vi "TriggerAndAveraging.vi"(7 "Channel":i32, 8 "error in (no error)":errorcluster, 11 "C4209 PNA":refnum<class "C4209 PNA.lvclass">) -> (0 "error out":errorcluster, 3 "C4209 PNA out":refnum<class "C4209 PNA.lvclass">)   [LabVIEW 2017, in "C4209 PNA.lvclass"]
uses:
  C4209 PNA.lvclass
  C4209 PNA.lvclass/C4209 PNA.ctl
  <instrlib>/CMT S2 Series VNA/CMT S2 Series VNA.lvlib
panel:
  # "do not input this here,\nbut at config time, for this application"
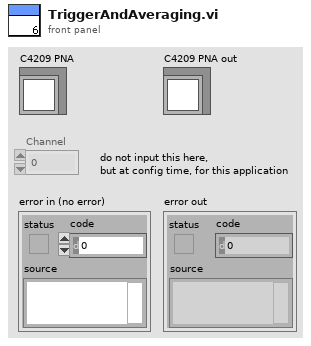
[diagram p1: front panel]
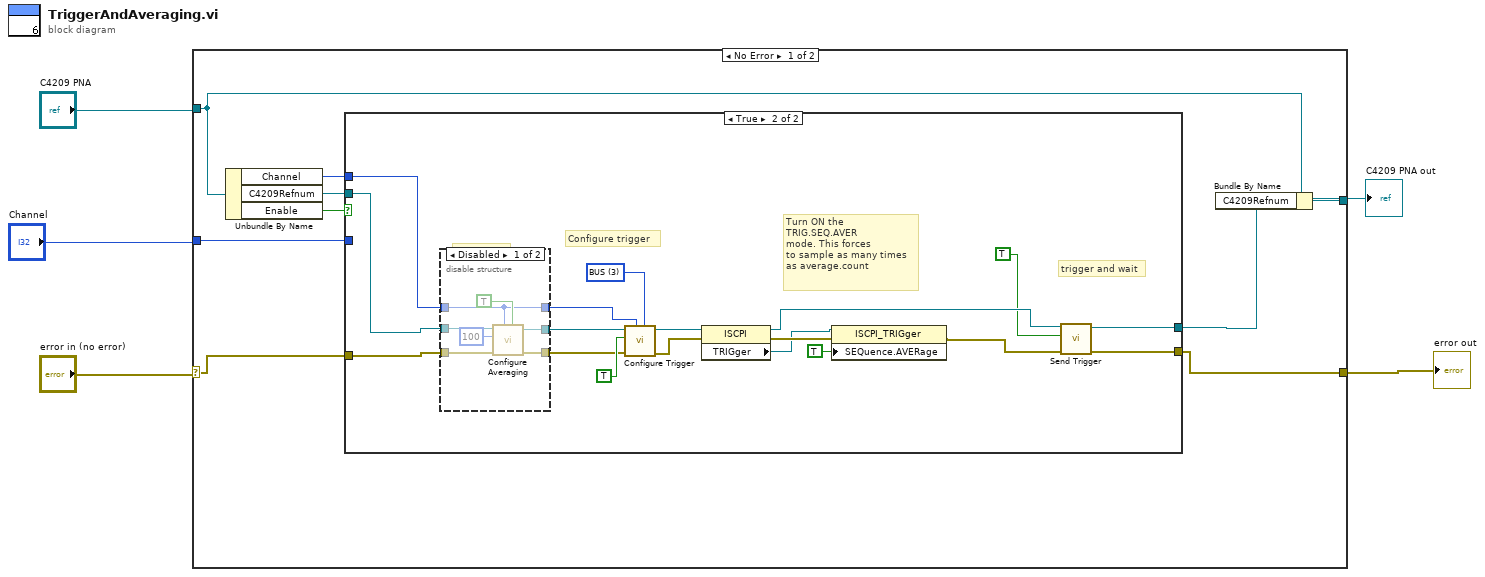
[diagram p0: block diagram]
diagram:
  n1 = case shown="No Error" "error in (no error)" {
    selector: "error in (no error)" -> [w13 w46]
    tunnel: [w12 w46] -> w4
    tunnel: [w11 w45] -> w2
    tunnel: "C4209 PNA" -> [w10 w45]
    tunnel: "Channel" -> [w8 _]
    frame No Error {
      n2 = Unbundle By Name(w10) -> ("Channel"=w6:i32, "C4209Refnum"=w14:refnum<k7>, "Enable"=w7:bool)
      n3 = case shown="True" w7 {
        tunnel: w14 -> [w16 w34]
        tunnel: w13 -> [w15 w33]
        tunnel: [w15 w32] -> w12
        tunnel: [w16 w31] -> w9
        tunnel: w8 -> [_ _]
        tunnel: w6 -> [_ w18]
        frame False {
        }
        frame True {
          w27 = u16 3 items=["Internal", "External", "Manual", "BUS"] ("Trigger Source (0: Internal)")
          # "trigger and wait"
          # "Turn ON the\nTRIG.SEQ.AVER\nmode. This forces\nto sample as many times\nas average.count"
          # "Configure trigger"
          n4 = disable-structure shown="Disabled" {
            disable-tunnel: w18 -> [w35 w42]
            disable-tunnel: w34 -> [w41 w44]
            disable-tunnel: w33 -> [w40 w43]
            disable-tunnel: [w39 w43] -> w21
            disable-tunnel: [w38 w44] -> w20
            disable-tunnel: [w35 w42] -> w17
            frame Disabled {
              # "delete this"
              n5 = call <instrlib>:"Configure Averaging.vi"("Averaging State (F: Off)"=TRUE, "Channel (1)"=w35, "error in (no error)"=w40, "Factor (16)"=100, "Reference in"=w41) -> ("error out"=w39:errorcluster, "Reference out"=w38:refnum<k7>)  [unwired: 5 in]
            }
            frame Enabled {
            }
          }
          n6 = call <instrlib>:"Configure Trigger.vi"("Trigger Source (0: Internal)"=w27, "Channel (1)"=w17, "error in (no error)"=w21, "Continuous Sweep (T: Enable)"=TRUE, "Reference in"=w20) -> ("error out"=w24:errorcluster, "Reference out"=w25:refnum<k7>)  [unwired: 5 in]
          n7 = property class="ISCPI"(reference=w25, error in=w24) -> (reference out=w23:refnum<k7>, error out=w30:errorcluster, "TRIGger"=w29:refnum<k7>)
          n8 = property class="ISCPI_TRIGger"(reference=w29, error in=w30, "SEQuence.AVERage"=TRUE) -> (error out=w22:errorcluster)  [unwired: 1 out]
          n9 = call <instrlib>:"Send Trigger.vi"("error in (no error)"=w22, "Wait for Sweep Completion (T: Wait)"=TRUE ("Continuous Sweep (T: Enable)"), "Reference in"=w23) -> ("error out"=w32:errorcluster, "Reference out"=w31:refnum<k7>)  [unwired: 7 in]
        }
      }
      n10 = Bundle By Name(cluster=w10, "C4209Refnum"=w9) -> (w11:refnum<class "C4209 PNA.lvclass">)
    }
    frame Error {
    }
  }
  "error out" <- w4
  "C4209 PNA out" <- w2
